vi "Constant-to-Constant Resampling.vi"() -> ()   [LabVIEW 2020]
doc: "This example demonstrates how to use zero padding to ensure the resampled signal occupies the same time span as the input signal."
uses:
  <vilib>/Analysis/2dsp.llb/Resample (constant to constant,single -channel).vi
  <vilib>/Analysis/NI_AALPro.lvlib
  <vilib>/Analysis/NI_AALBase.lvlib
panel:
  out "Constant-to-Constant Resampling (with padding zeros)":cluster{"t0":dbl, "dt":dbl, dbl[]}[](graph)
  in  "block length":i32=20
  in  "number of blocks":i32=10
  in  "dt":dbl=2.8 min=0.0
  in  "delay":dbl
  out "Constant-to-Constant Resampling (without padding zeros)":cluster{"t0":dbl, "dt":dbl, dbl[]}[](graph)
  # "Overview: Demonstrates how to pad with zeros to get a resampled signal of the same time span as the input signal.\nRequirements: LabVIEW Full Development System\nInstructions:\n1. Run the VI. \n2. Compare the different resampled signals with and without padding zeros before resampling. When zeros are padded to the input signal before resampling, the resampled signal will be the same time span as the input signal.\n3. Change other parameters and run the VI again."
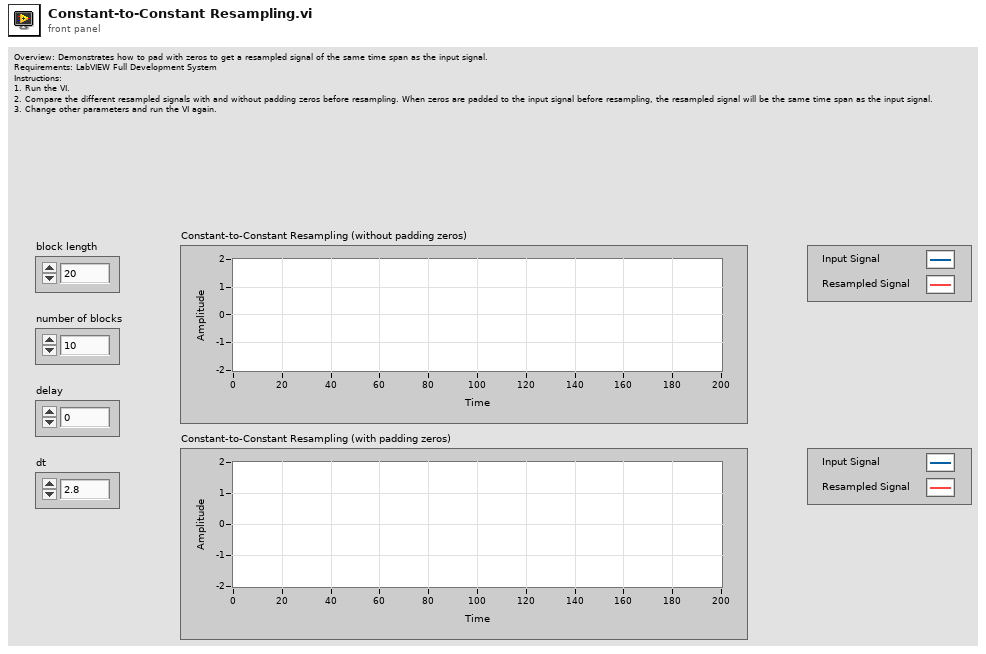
[diagram p1: front panel]
types:
  T1 = cluster{"frequency":dbl, "amplitude":dbl, "phase":dbl}[]
  T2 = cluster{"alias rejection (dB)":dbl, "normalized bandwidth":dbl}
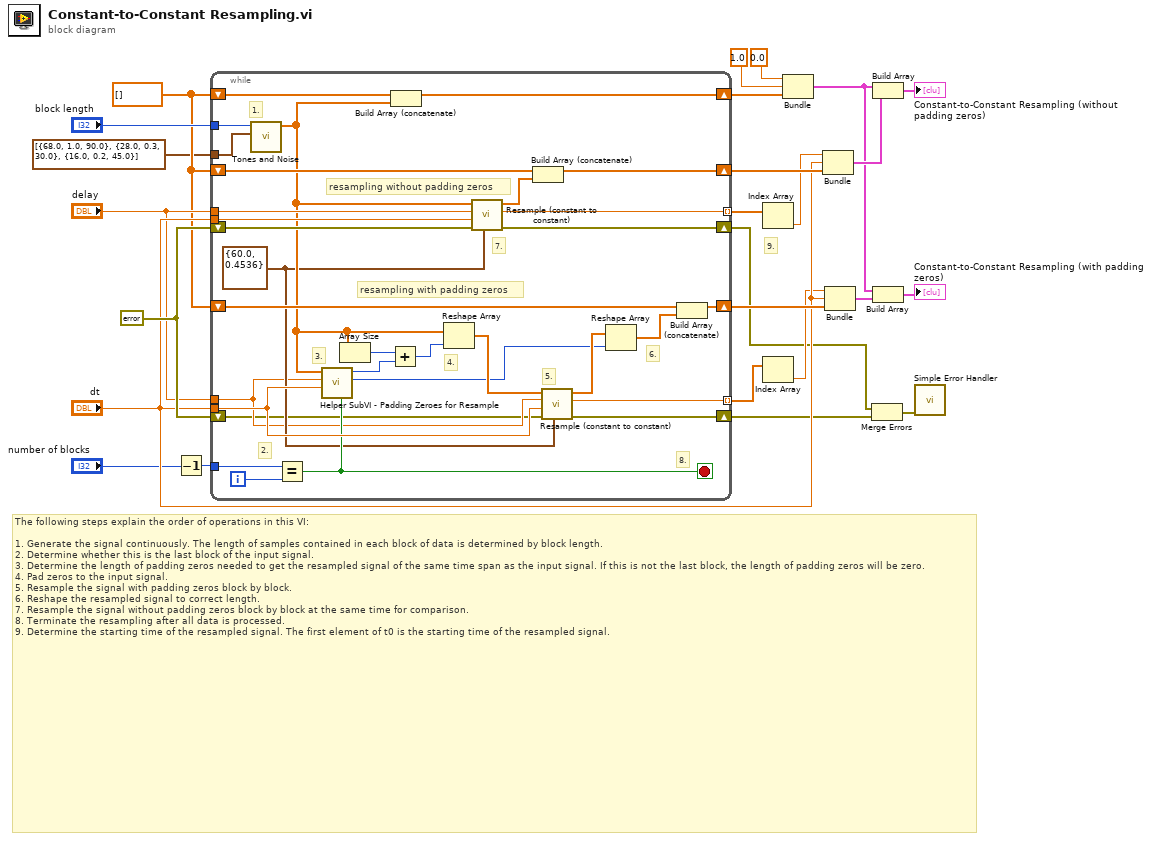
[diagram p0: block diagram]
diagram:
  w12 = errorcluster {"status"=FALSE, "code"=0, "source"=""} ("error out")
  w4 = dbl[] []
  # "9."
  # "The following steps explain the order of operations in this VI:\n\n1. Generate the signal continuously. The length of samples contained in each block of data is determined by block length.\n2. Determine whether this is the last block of the input signal.\n3. Determine the length of padding zeros needed to get the resampled signal of the same time span as the input signal. If this is not the last block, the length of padding zeros will be zero. \n4. Pad zeros to the input signal.\n5. Resample the signal with padding zeros block by block.\n6. Reshape the resampled signal to correct length.\n7. Resample the signal without padding zeros block by block at the same time for comparison.\n8. Terminate the resampling after all data is processed.\n9. Determine the starting time of the resampled signal. The first element of t0 is the starting time of the resampled signal."
  n1 = Decrement(x="number of blocks") -> (x-1=w2:i32)
  n2 = while {
    shift-right: [w55] -> w21
    shift-left: w4 -> [w56]
    shift-right: [w54] -> w25
    shift-left: w4 -> [w35]
    tunnel: "delay" -> [w47]
    shift-right: [w39] -> w5
    shift-left: w12 -> [w26]
    tunnel: [w41] -> w20 mode=indexing
    tunnel: "dt" -> [w46]
    tunnel: "block length" -> [w36]
    shift-right: [w42] -> w17
    shift-left: w4 -> [w43]
    shift-right: [w38] -> w6
    shift-left: w12 -> [w40]
    tunnel: "dt" -> [w37]
    tunnel: "delay" -> [w27]
    tunnel: [w33] -> w9 mode=indexing
    tunnel: w2 -> [w29]
    tunnel: T1 [{"frequency"=68.0, "amplitude"=1.0, "phase"=90.0}, {"frequency"=28.0, "amplitude"=0.3, "phase"=30.0}, {"frequency"=16.0, "amplitude"=0.2, "phase"=45.0}] ("tones") -> [w28]
    i -> [w31]
    stop <- w32 stop-if-true
    w30 = T2 {"alias rejection (dB)"=60.0, "normalized bandwidth"=0.4536} ("FIR filter specifications")
    # "7."
    # "resampling with padding zeros"
    # "resampling without padding zeros"
    # "8."
    # "6."
    # "5."
    # "4."
    # "3."
    # "2."
    # "1."
    n3 = call <vilib>:"Tones and Noise.vi"("tones"=w28, "samples"=w36) -> ("tones and noise"=w34:dbl[])  [unwired: 8 in, 1 out]
    n4 = Equal?(x=w29, y=w31) -> (x = y?=w32:bool)
    n5 = call "Helper SubVI - Padding Zeroes for Resample.vi"("padding zeroes?"=w32, "dt"=w46, "delay"=w27, "X"=w34) -> ("length of Y"=w48:i32, "length of padding zeros"=w51:i32)  [unwired: 6 in]
    n6 = Array Size(array=w34) -> (size(s)=w52:i32)
    n7 = Add(x=w52, y=w51) -> (x+y=w50:i32)
    n8 = Build Array (concatenate)(w35, w34) -> (w54:dbl[])
    n9 = Reshape Array(w34, w50) -> (w53:dbl[])
    n10 = call-poly <vilib>:"Resample (constant to constant).vi"("FIR filter specifications"=w30, "error in (no error)"=w40, "dt"=w37, "delay"=w47, "X"=w34) -> ("error out"=w38:errorcluster, "t0"=w41:dbl, "Y"=w45:dbl[])  [unwired: 4 in]
    n11 = Build Array (concatenate)(w56, w45) -> (w55:dbl[])
    n12 = call-poly <vilib>:"Resample (constant to constant).vi"("FIR filter specifications"=w30, "error in (no error)"=w26, "dt"=w46, "delay"=w27, "X"=w53) -> ("error out"=w39:errorcluster, "t0"=w33:dbl, "Y"=w49:dbl[])  [unwired: 4 in]
    n13 = Reshape Array(w49, w48) -> (w44:dbl[])
    n14 = Build Array (concatenate)(w43, w44) -> (w42:dbl[])
  }
  n15 = Index Array(array=w20) -> (element=w18:dbl)  [unwired: 1 in]
  n16 = Index Array(array=w9) -> (element=w8:dbl)  [unwired: 1 in]
  n17 = Bundle(0.0, 1.0, w25) -> (w16:cluster{dbl, dbl, dbl[]})  [unwired: 1 in]
  n18 = Bundle("t0"=w18, "dt"="dt", w21) -> (w22:cluster{"t0":dbl, "dt":dbl, dbl[]})  [unwired: 1 in]
  n19 = Bundle("t0"=w8, "dt"="dt", w17) -> (w15:cluster{"t0":dbl, "dt":dbl, dbl[]})  [unwired: 1 in]
  n20 = Merge Errors(w6, w5) -> (w7:errorcluster)
  n21 = Build Array(w16, w22) -> (→"Constant-to-Constant Resampling (without padding zeros)":cluster{"t0":dbl, "dt":dbl, dbl[]}[])
  n22 = Build Array(w16, w15) -> (→"Constant-to-Constant Resampling (with padding zeros)":cluster{"t0":dbl, "dt":dbl, dbl[]}[])
  n23 = call <vilib>:"Simple Error Handler.vi"("error in (no error)"=w7) -> ()  [unwired: 4 in, 5 out]
